vi "Send Configure Thermocouple [TC].vi"(7 "Message Priority (Normal)":T1=enum."Normal", 8 "error in (no error)":errorcluster, 9 "ref junc type (Internal)":i32(ring)=1 items=["Internal"=1, "Fixed"=2], 10 "thermocouple type (B)":i32(ring)=1 items=["B"=1, "C"=2, "D"=3, "E"=4, "G"=5, "J"=6, "K"=7, "N"=8, "R"=9, "S"=10, "T"=11, "U"=12, "V"=13], 11 "Message Enqueuer":refnum<class "Message Enqueuer.lvclass">) -> (0 "error out":errorcluster, 3 "Message Enqueuer out":refnum<class "Message Enqueuer.lvclass">)   [LabVIEW 2013, in "CS++DMM.lvlib" / "Configure Thermocouple [TC] Msg.lvclass"]
doc: "This VI sends the message to an actor."
uses:
  Configure Thermocouple [TC] Msg.lvclass
  <vilib>/ActorFramework/Message Enqueuer/Message Enqueuer.lvclass
  <vilib>/ActorFramework/Message Enqueuer/Message Priority.ctl
  Configure Thermocouple [TC] Msg.lvclass/Configure Thermocouple [TC] Msg.ctl
  <vilib>/ActorFramework/Message Enqueuer/Message Enqueuer.lvclass/Message Enqueuer.ctl
  <vilib>/ActorFramework/Message Priority Queue/Priority Enqueue.vi
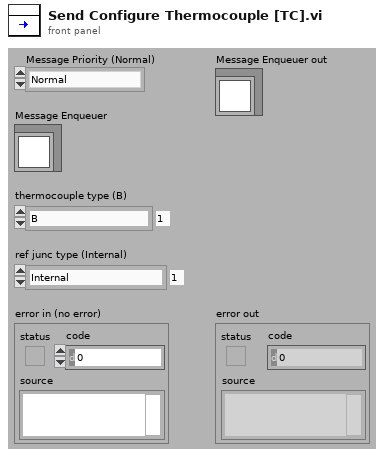
[diagram p1: front panel]
types:
  T1 = typedef "Actor Framework.lvlib/Message Enqueuer.lvclass/Message Priority.ctl" = enum16{"Low", "Normal", "High"}
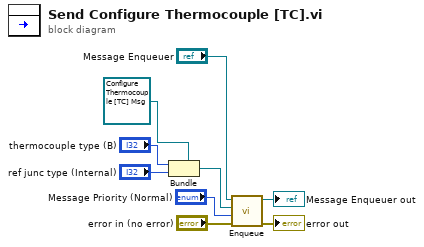
[diagram p0: block diagram]
diagram:
  n1 = Bundle(cluster=refnum<class "Configure Thermocouple [TC] Msg.lvclass"> refnum ("Object"), "thermocouple type (B)", "ref junc type (Internal)") -> (w5:refnum<class "Configure Thermocouple [TC] Msg.lvclass">)
  n2 = call <vilib>:"Enqueue.vi"("error in (no error)"="error in (no error)", "Message Priority (Normal)"="Message Priority (Normal)", "Message"=w5, "Message Enqueuer in"="Message Enqueuer") -> ("error out"=→"error out":errorcluster, "Message Enqueuer out"=→"Message Enqueuer out":refnum<class "Message Enqueuer.lvclass">)  [unwired: 6 in]
